vi "Set External Network Present.vi"(8 "error in (no error)":errorcluster, 11 "QPA Measurement in":refnum<class "QPA Measurement.lvclass">) -> (0 "error out":errorcluster, 3 "QPA Measurement out":refnum<class "QPA Measurement.lvclass">)   [LabVIEW 2016, in "QPA Measurement.lvlib" / "QPA Measurement.lvclass"]
uses:
  QPA Measurement.lvclass
  C:/Projects/STS/Common/Sequence Automation/Plugins/Measurement Interface.lvlibp/Measurement Interface.lvclass
  QPA Measurement.lvclass/QPA Measurement.ctl
  Protected Methods/Read External Network Step.vi
  Protected Methods/Read Measurement Name.vi
  Protected Methods/Write External Network Present.vi
  Plugins/Measurement Interface.lvlibp/Private Methods/Measurement Parameters/Read Measurement Parameters.vi
  Plugins/String Database.lvlibp/String Database.lvclass
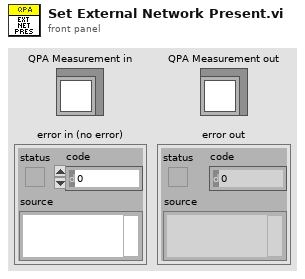
[diagram p1: front panel]
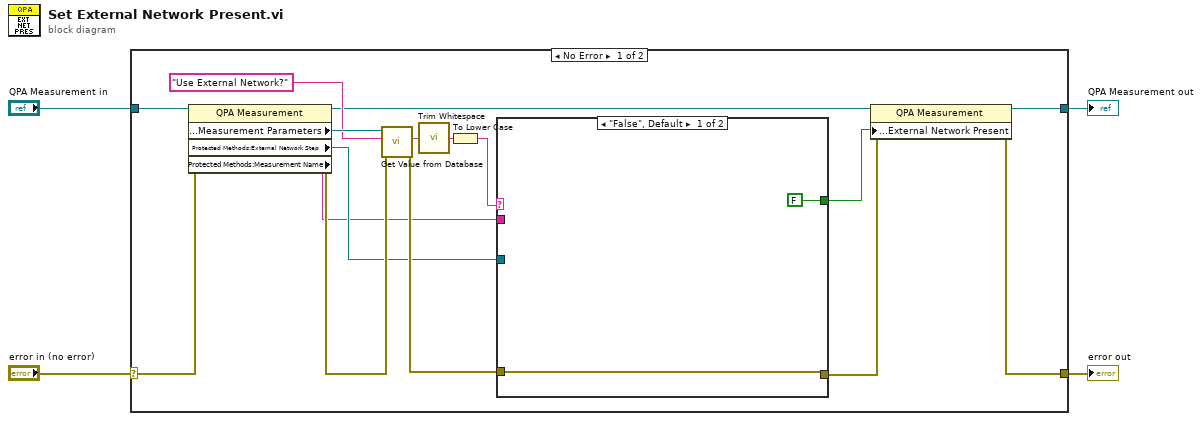
[diagram p0: block diagram]
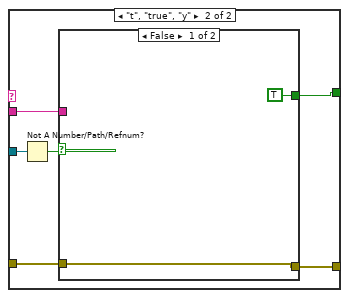
[diagram p2: hidden frame]
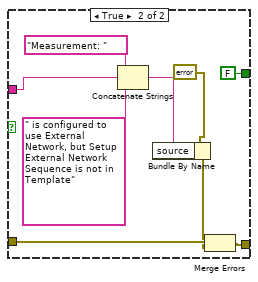
[diagram p3: hidden frame]
diagram:
  n1 = case shown="No Error" "error in (no error)" {
    selector: "error in (no error)" -> [w20 w41]
    tunnel: [w14 w41] -> w3
    tunnel: [w12 w40] -> w1
    tunnel: "QPA Measurement in" -> [w19 w40]
    frame No Error {
      n2 = property class="QPA Measurement"(reference=w19, error in=w20) -> (reference out=w13:refnum<class "QPA Measurement.lvclass">, error out=w17:errorcluster, "Protected Methods:Measurement Parameters"=w18:refnum<class "String Database.lvclass">, "Protected Methods:External Network Step"=w8:refnum<k7>, "Protected Methods:Measurement Name"=w6:string)
      n3 = call "Get Value from Database.vi"("error in (no error)"=w17, "Entry Name"="Use External Network?", "Message in"=w18) -> ("error out"=w9:errorcluster, "Entry Value"=w15:string)  [unwired: 5 in, 2 out]
      n4 = call <vilib>:"Trim Whitespace.vi"("string"=w15) -> ("trimmed string"=w10:string)  [unwired: 1 in]
      n5 = To Lower Case(string=w10) -> (all lower case string=w5:string)
      n6 = case shown="\"False\", Default" w5 {
        tunnel: [FALSE w23] -> w11
        tunnel: w9 -> [w21 w26]
        tunnel: w8 -> [_ w28]
        tunnel: [w21 w25] -> w7
        tunnel: w6 -> [_ w24]
        frame "False", Default {
        }
        frame "t", "true", "y" {
          n7 = Not A Number/Path/Refnum?(number/path/refnum=w28) -> (NaN/Path/Refnum?=w27:bool)
          n8 = case shown="False" w27 {
            tunnel: w26 -> [w30 w39]
            tunnel: [w30 w37] -> w25
            tunnel: w24 -> [_ w35]
            tunnel: [TRUE FALSE] -> w23
            frame False {
            }
            frame True {
              n9 = Concatenate Strings("Measurement: " ("source"), w35, " is configured to use External Network, but Setup External Network Sequence is not in Template" ("source")) -> (w33:string)
              n10 = Bundle By Name(cluster=errorcluster {"status"=TRUE, "code"=8555, "source"=""} ("error constant"), "source"=w33) -> (w32:errorcluster)
              n11 = Merge Errors(w39, w32) -> (w37:errorcluster)
            }
          }
        }
      }
      n12 = property class="QPA Measurement"(reference=w13, error in=w7, "Protected Methods:External Network Present"=w11) -> (reference out=w12:refnum<class "QPA Measurement.lvclass">, error out=w14:errorcluster)
    }
    frame Error {
    }
  }
  "error out" <- w3
  "QPA Measurement out" <- w1
